vi "Send to Home.vi"(7 "from local":bool=TRUE, 8 "error in (no error)":errorcluster, 10 "position":dbl[](array[numeric]), 11 "Mototr Queue in":refnum<queue>) -> (0 "error out":errorcluster, 3 "Mototr Queue out":refnum<queue>)   [LabVIEW 2020]
uses:
  Message Queue/Message Cluster.ctl
  PCT FGV CMD.ctl
  Message Queue/Message Queue.lvlib
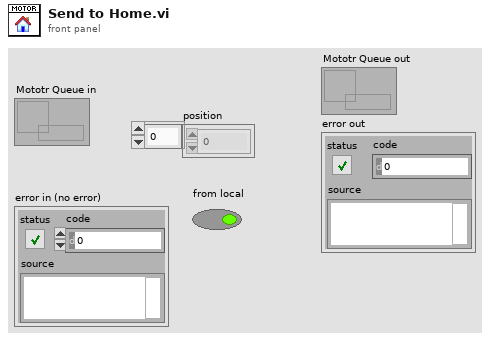
[diagram p1: front panel]
types:
  T1 = typedef "PCT FGV CMD.ctl" = enum16{"INIT", "GET", "SET"}
  T2 = cluster{"Type CMD":string, "Mode CMD":string, "Main CMD":string}
  T3 = cluster{"position[0]":dbl, "position[1]":dbl, "position[2]":dbl, "position[3]":dbl}
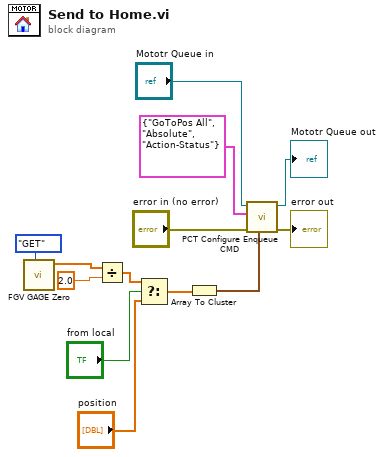
[diagram p0: block diagram]
diagram:
  n1 = call "FGV GAGE Zero.vi"("CMD"=PCT_FGV_CMD."GET") -> ("output"=w2:dbl[])  [unwired: 9 in, 1 out]
  n2 = Divide(x=w2, y=2.0 ("Numeric")) -> (x/y=w1:dbl[])
  n3 = Select(t=w1, s="from local", f="position") -> (s? t:f=w4:dbl[])
  n4 = Array To Cluster(array=w4) -> (cluster=w7:T3)
  n5 = call "PCT Configure Enqueue CMD.vi"("Parameter Data"=w7, "error in (no error)"="error in (no error)", "CMD"=T2 {"Type CMD"="GoToPos All", "Mode CMD"="Absolute", "Main CMD"="Action-Status"}, "CMD Queue in"="Mototr Queue in") -> ("error out"=→"error out":errorcluster, "CMD Queue out"=→"Mototr Queue out":refnum<queue>)  [unwired: 5 in, 1 out]
